vi "main.vi"() -> ()   [LabVIEW 2019]
panel:
  out "IVC (Torr)":dbl
  in  "milliseconds to wait":u32=1000
  out "Numeric":i32
  in  "stop":bool
  out "return count":u32
  out "concatenated string":string
  out "error out":errorcluster
  in  "error in":errorcluster
  out "IVC":string
  out "read buffer":string
  in  "VISA resource name":refnum<visa-resource-name>
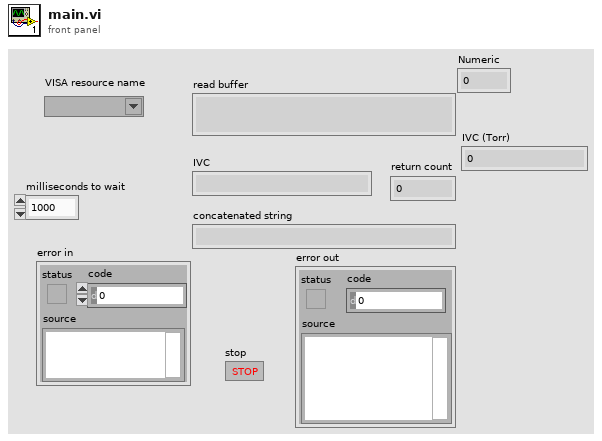
[diagram p1: front panel]
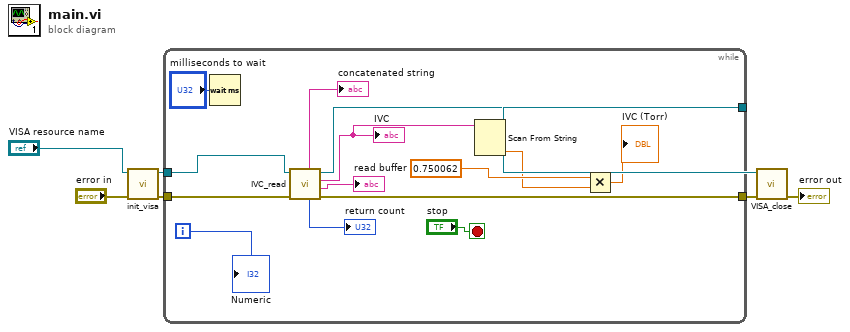
[diagram p0: block diagram]
diagram:
  n1 = call "init_visa.vi"("error in"="error in", "VISA resource name"="VISA resource name") -> ("error out"=w4:errorcluster, "VISA resource name out"=w5:refnum<visa-resource-name>)  [unwired: 8 in]
  n2 = while {
    tunnel: w5 -> [w18]
    tunnel: w4 -> [w17]
    tunnel: [w16] -> w3
    tunnel: [w15] -> w2
    i -> [w14]
    stop <- "stop" stop-if-true
    n3 = Wait (ms)(milliseconds to wait="milliseconds to wait") -> ()  [unwired: 1 out]
    n4 = call "IVC_read.vi"("error in (no error)"=w17, "VISA Refnum in"=w18) -> ("error out"=w16:errorcluster, "read buffer"=→"read buffer":string, "IVC"=w10:string, "VISA Refnum out"=w15:refnum<visa-resource-name>, "return count"=→"return count":u32, "concatenated string"=→"concatenated string":string)  [unwired: 4 in]
    "IVC" <- w10
    n5 = Scan From String(input string=w10) -> (output 1=w9:dbl)  [unwired: 4 in, 3 out]
    n6 = Multiply(x=0.750062 ("y"), y=w9) -> (x*y=→"IVC (Torr)":dbl)
    "Numeric" <- w14
  }
  n7 = call "VISA_close.vi"("error in (no error)"=w3, "VISA resource name"=w2) -> ("error out"=→"error out":errorcluster)  [unwired: 9 in]
